vi "rd_initialHeader.vi"(4 "actualTimeIndex":i32, 6 "actualDataIndex":i32, 8 "error in (no error)":errorcluster, 9 "TimeColumnMode":T1, 10 "column index":i32, 11 "header":string) -> (0 "error out":errorcluster, 1 "actualTimeIndex":i32, 2 "actualDataIndex":i32, 3 "header out":string)   [LabVIEW 2020, in "NI_ExcelFile.lvlib"]
uses:
  <vilib>/express/express shared/NI_ExcelFile/NI_ExcelFile.lvlib
  <vilib>/express/express shared/NI_ExcelFile/Ctrls/TimeColumnMode.ctl
panel:
  in  "default time header":string="Time"
  in  "default data header":string="Untitled"
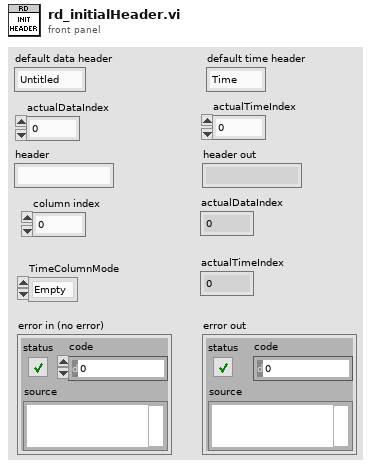
[diagram p1: front panel]
types:
  T1 = typedef "NI_ExcelFile.lvlib/TimeColumnMode.ctl" = enum16{"Empty", "OnePerCh", "One"}
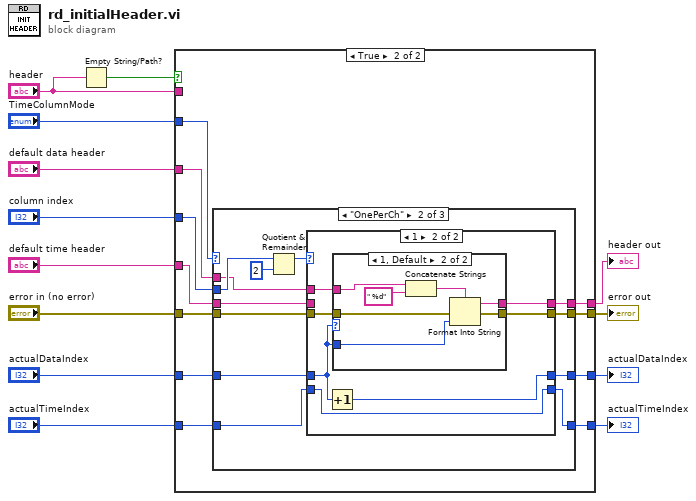
[diagram p0: block diagram]
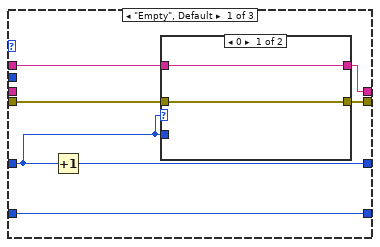
[diagram p3: hidden frame]
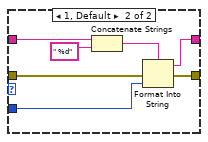
[diagram p4: hidden frame]
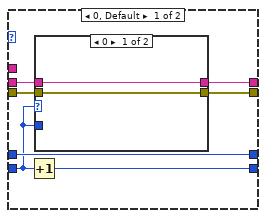
[diagram p5: hidden frame]
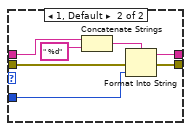
[diagram p6: hidden frame]
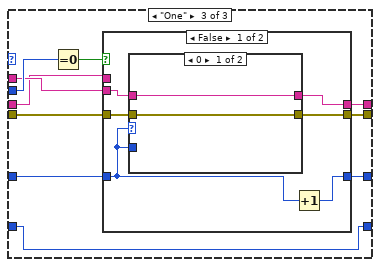
[diagram p8: hidden frame]
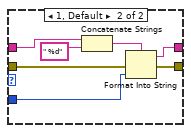
[diagram p9: hidden frame]
diagram:
  n1 = Empty String/Path?(string/path="header") -> (empty?=w7:bool)
  n2 = case shown="True" w7 {
    tunnel: "TimeColumnMode" -> [_ w28]
    tunnel: "column index" -> [_ w27]
    tunnel: "error in (no error)" -> [w17 w26]
    tunnel: [w17 w25] -> w8
    tunnel: [w16 w24] -> w9
    tunnel: "header" -> [w16 _]
    tunnel: "actualDataIndex" -> [w15 w23]
    tunnel: [w15 w22] -> w5
    tunnel: "actualTimeIndex" -> [w14 w21]
    tunnel: [w14 w20] -> w3
    tunnel: "default data header" -> [_ w19]
    tunnel: "default time header" -> [_ w18]
    frame False {
    }
    frame True {
      n3 = case shown="\"OnePerCh\"" w28 {
        tunnel: w27 -> [_ w54 w97]
        tunnel: [w33 w51 w94] -> w24
        tunnel: w26 -> [w35 w53 w96]
        tunnel: [w34 w52 w95] -> w25
        tunnel: w23 -> [w30 w50 w93]
        tunnel: [w32 w49 w92] -> w22
        tunnel: w21 -> [w31 w48 w91]
        tunnel: [w31 w47 w91] -> w20
        tunnel: w19 -> [w29 w46 w90]
        tunnel: w18 -> [_ w45 w89]
        frame "Empty", Default {
          n4 = Increment(x=w30) -> (x+1=w32:i32)
          n5 = case shown="0" w30 {
            tunnel: w35 -> [w36 w44]
            tunnel: [w36 w43] -> w34
            tunnel: [w37 w42] -> w33
            tunnel: w30 -> [_ w41]
            tunnel: w29 -> [w37 w40]
            frame 0 {
            }
            frame 1, Default {
              n6 = Concatenate Strings(w40, " %d" ("format string")) -> (w38:string)
              n7 = Format Into String(format string=w38, error in=w44, w41) -> (resulting string=w42:string, error out=w43:errorcluster)  [unwired: 1 in]
            }
          }
        }
        frame "OnePerCh" {
          n8 = Quotient & Remainder(x=w54, y=2) -> (x-y*floor(x/y)=w55:i32)  [unwired: 1 out]
          n9 = case shown="1" w55 {
            tunnel: [w63 w79] -> w51
            tunnel: w53 -> [w62 w78]
            tunnel: [w61 w77] -> w52
            tunnel: w50 -> [w60 w74]
            tunnel: [w60 w76] -> w49
            tunnel: w48 -> [w58 w75]
            tunnel: [w59 w75] -> w47
            tunnel: w46 -> [_ w73]
            tunnel: w45 -> [w57 _]
            frame 0, Default {
              n10 = Increment(x=w58) -> (x+1=w59:i32)
              n11 = case shown="0" w58 {
                tunnel: [w65 w72] -> w63
                tunnel: w62 -> [w64 w71]
                tunnel: [w64 w70] -> w61
                tunnel: w58 -> [_ w69]
                tunnel: w57 -> [w65 w68]
                frame 0 {
                }
                frame 1, Default {
                  n12 = Concatenate Strings(w68, " %d" ("format string")) -> (w66:string)
                  n13 = Format Into String(format string=w66, error in=w71, w69) -> (resulting string=w72:string, error out=w70:errorcluster)  [unwired: 1 in]
                }
              }
            }
            frame 1 {
              n14 = Increment(x=w74) -> (x+1=w76:i32)
              n15 = case shown="1, Default" w74 {
                tunnel: [w81 w88] -> w79
                tunnel: w78 -> [w80 w87]
                tunnel: [w80 w86] -> w77
                tunnel: w74 -> [_ w85]
                tunnel: w73 -> [w81 w84]
                frame 0 {
                }
                frame 1, Default {
                  n16 = Concatenate Strings(w84, " %d" ("format string")) -> (w82:string)
                  n17 = Format Into String(format string=w82, error in=w87, w85) -> (resulting string=w88:string, error out=w86:errorcluster)  [unwired: 1 in]
                }
              }
            }
          }
        }
        frame "One" {
          n18 = Equal To 0?(x=w97) -> (x = 0?=w98:bool)
          n19 = case shown="False" w98 {
            tunnel: [w104 w114] -> w94
            tunnel: w96 -> [w103 w115]
            tunnel: [w99 w115] -> w95
            tunnel: w93 -> [w101 w116]
            tunnel: [w102 w116] -> w92
            tunnel: w90 -> [w100 _]
            tunnel: w89 -> [_ w114]
            frame False {
              n20 = case shown="0" w101 {
                tunnel: [w106 w113] -> w104
                tunnel: w103 -> [w105 w112]
                tunnel: w101 -> [_ w110]
                tunnel: w100 -> [w106 w109]
                tunnel: [w105 w111] -> w99
                frame 0 {
                }
                frame 1, Default {
                  n21 = Concatenate Strings(w109, " %d" ("format string")) -> (w107:string)
                  n22 = Format Into String(format string=w107, error in=w112, w110) -> (resulting string=w113:string, error out=w111:errorcluster)  [unwired: 1 in]
                }
              }
              n23 = Increment(x=w101) -> (x+1=w102:i32)
            }
            frame True {
            }
          }
        }
      }
    }
  }
  "header out" <- w9
  "error out" <- w8
  "actualDataIndex" <- w5
  "actualTimeIndex" <- w3
